vi "Day 3 - part two.vi"() -> ()   [LabVIEW 2023]
panel:
  out "sum 2":dbl
  out "Array 3":string[](array[string])
  out "array":string[](array[string])
  in  "input":string="WjmsdnddnmQPZPPJPL\nbQllTtpBlgwtrbbCwfZcfSFPSfLCSF\nGgVgQrlpphBGrlVGgTtsRHRWVRMzRdVsqdnDnV\nMMTcbpnfNGQbMjgsRwSzRptRzz\nlPqCCqQdQqQmCPRzRVSwtzgqqwqR\nlrDdllPdBWdDFQFnMbDNDn\nFldWTldlpBSLzvpnpSTpWbDhbHNDPHhJcNHNDwbH\nqVCGQRGrrgMQrJhPNchgvgJhNc\nfrjGfMrGQMjsRrRQjvQGmrQQszTTpSLBznlzBlLLSBLLSZTn\nTPZZZMTTbNTZNtTlTbjPVRVGzpGQLLzdGgmslhzSzgLzQh\nwrfwDDvcnFvCfrrSQsmzGGQQdndsGg\nqfHwHCqCqCrFJrcBHCCJRmWTRTmVMttjRjRHZMNV\nvpbqnzbPmWLFjFLBnjZg\nNltQcCClQlcGQGtMTCRdGTGBFZRLZjFFZZhBPLrFHZFjHf\nlMtlGMwMsCCNlTwtsCPzzmPmmVpmpWqVWsWz\nVmWVSchSrScGtwlVtBnwBVFF\nRZZPRNpPCLZvZPZNCLbQPZNBFtttmwBMTMTtttCwtgwBgl\nRNNmPvbQQjPRQQNNHpN..."
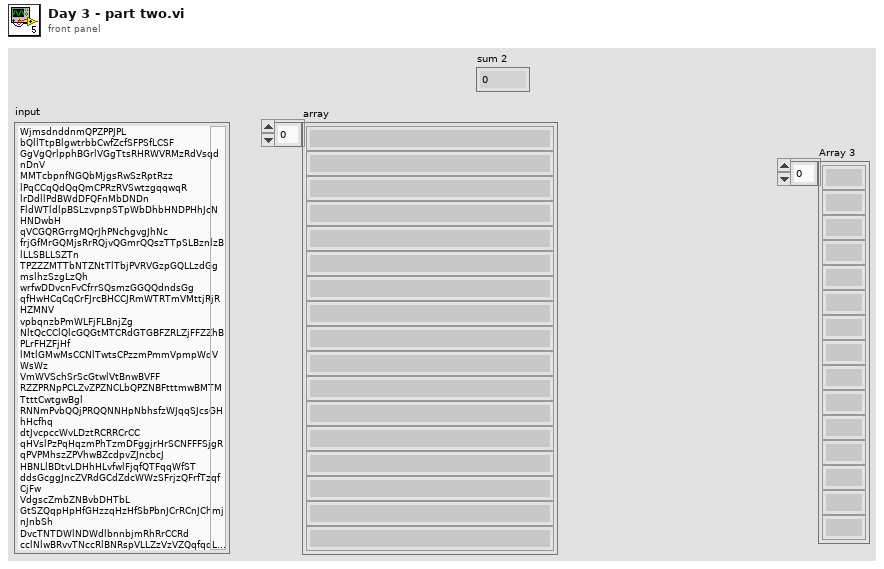
[diagram p1: front panel]
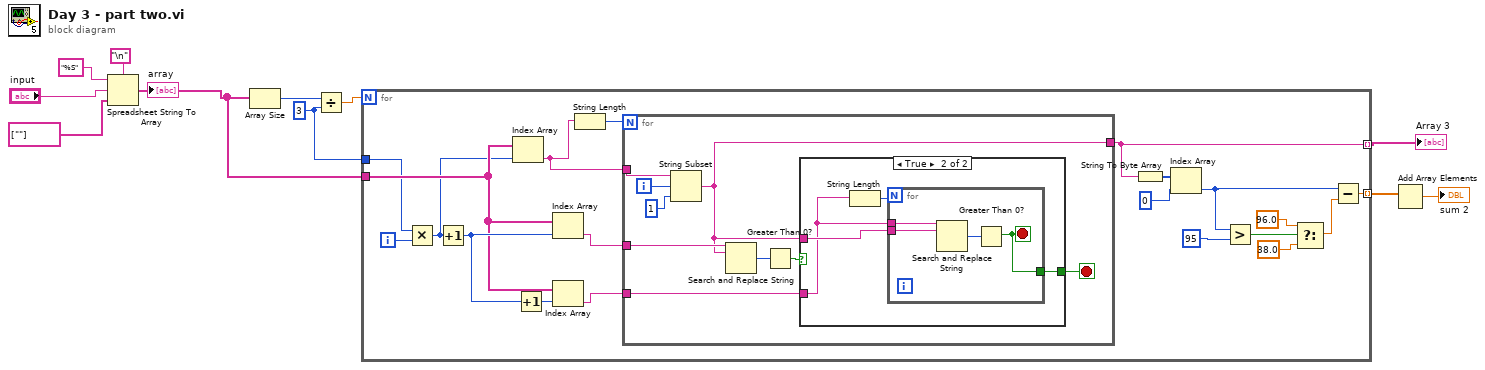
[diagram p0: block diagram]
diagram:
  w1 = 3 ("y")
  n1 = Spreadsheet String To Array(delimiter (Tab)="\n", format string="%S", spreadsheet string="input", array type (2D Dbl)=string[] [""]) -> (array=w7:string[])
  "array" <- w7
  n2 = Array Size(array=w7) -> (size(s)=w4:i32)
  n3 = Divide(x=w4, y=w1) -> (x/y=w5:dbl)
  n4 = for {
    N: w5 -> [_]
    tunnel: w7 -> [w26]
    tunnel: [w16] -> w6 mode=indexing
    tunnel: [w14] -> w3 mode=indexing
    tunnel: w1 -> [w12]
    i -> [w15]
    n5 = Multiply(x=w12, y=w15) -> (x*y=w13:i32)
    n6 = Increment(x=w13) -> (x+1=w27:i32)
    n7 = Index Array(array=w26, index=w13) -> (element=w30:string)
    n8 = Increment(x=w27) -> (x+1=w28:i32)
    n9 = Index Array(array=w26, index=w27) -> (element=w29:string)
    n10 = Index Array(array=w26, index=w28) -> (element=w25:string)
    n11 = String Length(string=w30) -> (length=w31:i32)
    n12 = for {
      N: w31 -> [_]
      tunnel: w30 -> [w39]
      tunnel: w29 -> [w40]
      tunnel: [w33] -> w16
      tunnel: w25 -> [w34]
      i -> [w38]
      stop <- w32 stop-if-true
      n13 = String Subset(string=w39, offset (0)=w38, length (rest)=1 ("length (rest)")) -> (substring=w33:string)
      n14 = Search and Replace String(input string=w40, search string=w33) -> (number of replacements=w36:i32)  [unwired: 6 in, 3 out]
      n15 = Greater Than 0?(x=w36) -> (x > 0?=w35:bool)
      n16 = case shown="True" w35 {
        tunnel: w34 -> [_ w41]
        tunnel: w33 -> [_ w44]
        tunnel: [_ w43] -> w32
        frame False {
        }
        frame True {
          n17 = String Length(string=w41) -> (length=w42:i32)
          n18 = for {
            N: w42 -> [_]
            tunnel: w41 -> [w47]
            tunnel: w44 -> [w46]
            tunnel: [w45] -> w43
            stop <- w45 stop-if-true
            n19 = Search and Replace String(input string=w47, search string=w46) -> (number of replacements=w48:i32)  [unwired: 6 in, 3 out]
            n20 = Greater Than 0?(x=w48) -> (x > 0?=w45:bool)
          }
        }
      }
    }
    n21 = String To Byte Array(string=w16) -> (unsigned byte array=w23:u8[])
    n22 = Index Array(array=w23, index=0) -> (element=w24:u8)
    n23 = Greater?(x=w24, y=u8 95) -> (0:w19:bool)
    n24 = Select(t=96.0, s=w19, f=38.0) -> (s? t:f=w22:dbl)
    n25 = Subtract(x=w24, y=w22) -> (x-y=w14:dbl)
  }
  "Array 3" <- w6
  n26 = Add Array Elements(numeric array=w3) -> (sum=→"sum 2":dbl)
